vi "PPS_TRAJECTORY_EXECUTE_REL.vi"(8 "Init":bool, 10 "End Relative\nOrientation Deg":dbl, 11 "Gyro Heading\nRAD":dbl) -> (0 "AtReference":bool, 3 "Chassis Velocity Target SI":T7 {"vOmega" format="%10.3f"; "vY" format="%10.3f"; "vX" format="%10.3f"})   [LabVIEW 2019]
uses:
  <vilib>/Rock Robotics/WPI/ThirdParty/JAS_Junk/TrajLib/Trajectory_Library.lvlib
  PPR_TRAJECTORY_GLOBALS.vi
  <vilib>/Rock Robotics/WPI/ThirdParty/MJansen/PathPlanner/PathPlanner24.lvlib
  <vilib>/Rock Robotics/WPI/ThirdParty/JAS_Junk/TrajLib/TypeDef/CHASSIS_SPEEDS.ctl
  <vilib>/Rock Robotics/WPI/ThirdParty/JAS_Junk/TrajLib/TypeDef/TRANSLATION2D.ctl
  <vilib>/Rock Robotics/WPI/ThirdParty/JAS_Junk/TrajLib/TypeDef/ROTATION2D.ctl
  <vilib>/Rock Robotics/WPI/ThirdParty/MJansen/PathPlanner/TypeDef/PathPlannerTrajectory.ctl
  <vilib>/Rock Robotics/WPI/ThirdParty/MJansen/PathPlanner/TypeDef/PathPlannerTrajectoryState.ctl
  <vilib>/Rock Robotics/WPI/ThirdParty/MJansen/PathPlanner/TypeDef/PathPlannerPathConstraints.ctl
panel:
  out "PathPlannerTrajectory":T1 {"States"."TargetHolonomicRotation"."SIN" format="%13.4f"; "States"."TargetHolonomicRotation"."COS" format="%13.4f"; "States"."TargetHolonomicRotation"."VALUE" format="%13.4f"; "States"."Heading"."SIN" format="%13.4f"; "States"."Heading"."COS" format="%13.4f"; "States"."Heading"."VALUE" format="%13.4f"; "States"."PositionMeters"."Y" format="%14.3f"; "States"."PositionMeters"."X" format="%14.3f"}
  in  "Robot Params":T6={"Max Module Speed M/S"=3.2, "Drive Base Radius M"=0.6}
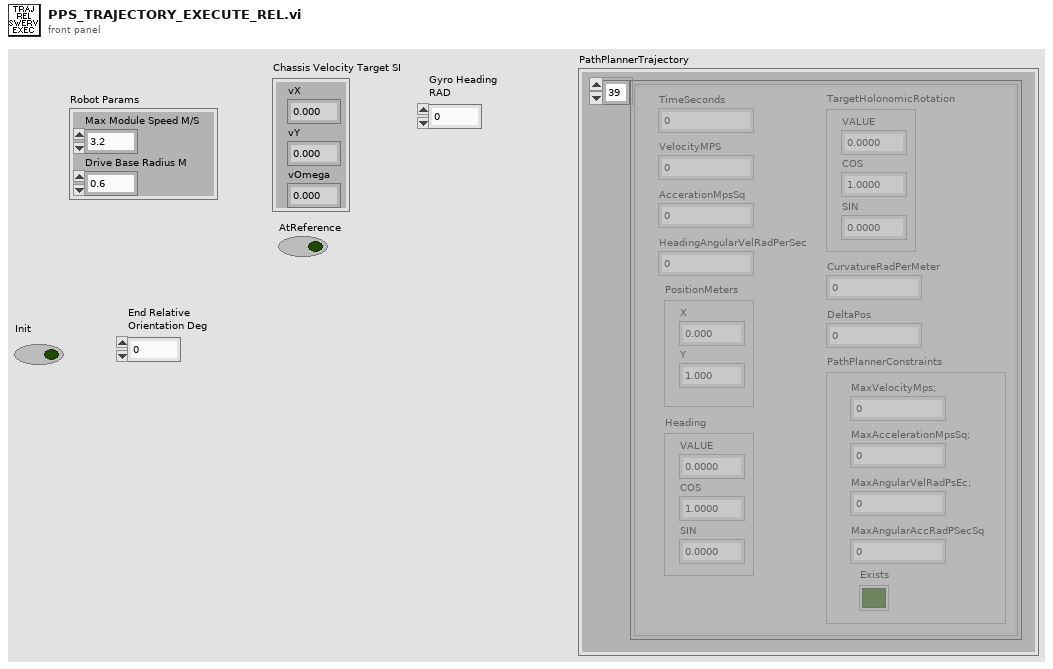
[diagram p1: front panel]
types:
  T1 = typedef "PathPlanner24.lvlib/PathPlannerTrajectory.ctl" = cluster{"States":T2[]}
  T2 = typedef "PathPlanner24.lvlib/PathPlannerTrajectoryState.ctl" = cluster{"TimeSeconds":dbl, "VelocityMPS":dbl, "AccerationMpsSq":dbl, "HeadingAngularVelRadPerSec":dbl, "PositionMeters":T3, "Heading":T4, "TargetHolonomicRotation":T4, "CurvatureRadPerMeter":dbl, "PathPlannerConstraints":T5, "DeltaPos":dbl}
  T3 = typedef "Trajectory_Library.lvlib/TRANSLATION2D.ctl" = cluster{"X":dbl, "Y":dbl}
  T4 = typedef "Trajectory_Library.lvlib/ROTATION2D.ctl" = cluster{"VALUE":dbl, "COS":dbl, "SIN":dbl}
  T5 = typedef "PathPlanner24.lvlib/PathPlannerPathConstraints.ctl" = cluster{"MaxVelocityMps;":dbl, "MaxAccelerationMpsSq;":dbl, "MaxAngularVelRadPsEc;":dbl, "MaxAngularAccRadPSecSq":dbl, "Exists":bool}
  T6 = cluster{"Max Module Speed M/S":dbl, "Drive Base Radius M":dbl}
  T7 = typedef "Trajectory_Library.lvlib/CHASSIS_SPEEDS.ctl" = cluster{"vX":dbl, "vY":dbl, "vOmega":dbl}
  T8 = typedef "Trajectory_Library.lvlib/DIFF_DRIVE_KINEMATICS.ctl" = cluster{"TrackWidth_Meters":dbl}
  T9 = typedef "Trajectory_Library.lvlib/POSE2D.ctl" = cluster{"TRANSLATION":T3, "ROTATION":T4}
  T10 = typedef "Trajectory_Library.lvlib/PID_TUNING.ctl" = cluster{"Kp":dbl, "Ki":dbl, "Kd":dbl, "MaximumIntegral":dbl, "MinimumIntegral":dbl}
  T11 = typedef "Trajectory_Library.lvlib/PROFILED_PID_CONTROLLER.ctl" = cluster{"Controller":T12, "Goal":T13, "Setpoint":T13, "Constraint":T14}
  T12 = typedef "Trajectory_Library.lvlib/PID_CONTROLLER.ctl" = cluster{"Kp":dbl, "Ki":dbl, "Kd":dbl, "Period":dbl, "Max_Integral":dbl, "Min_Integral":dbl, "Max_Input":dbl, "Min_Input":dbl, "Continuous":bool, "PositionError":dbl, "VelocityError":dbl, "PrevError":dbl, "TotalError":dbl, "PositionTolerance":dbl, "VelocityTolerance":dbl, "SetPoint":dbl, "Kf":dbl, "Prev_Deriv":dbl, "Prev_Deriv 2":dbl, "DerivativeFilter":bool, "Min_Output":dbl, "Max_Output":dbl, "Prev_F_P":dbl, "Prev_F_P_2":dbl, "AntiWindupActive":bool, "Measurement":dbl}
  T13 = typedef "Trajectory_Library.lvlib/TRAPEZOID_PROFILE_STATE.ctl" = cluster{"Position":dbl, "Velocity":dbl}
  T14 = typedef "Trajectory_Library.lvlib/TRAPEZOID_PROFILE_CONSTRAINT.ctl" = cluster{"MaxVelocity":dbl, "MaxAcceleration":dbl}
  T15 = typedef "Trajectory_Library.lvlib/HOLONOMIC_PACK_TUNING.ctl" = cluster{"X PID Tuning":T10, "Y PID Tuning":T10, "thetaProfiledPID_CTRL":T11}
  T16 = typedef "Trajectory_Library.lvlib/HOLONOMIC_DRV_CTRL.ctl" = cluster{"poseTolerance":T9, "poseError":T9, "Enabled":bool, "PID_xCtrl":T12, "PID_yCtrl":T12, "PROF_PID_thetaCtrl":T11, "RotationError":T4, "FirstRun":bool}
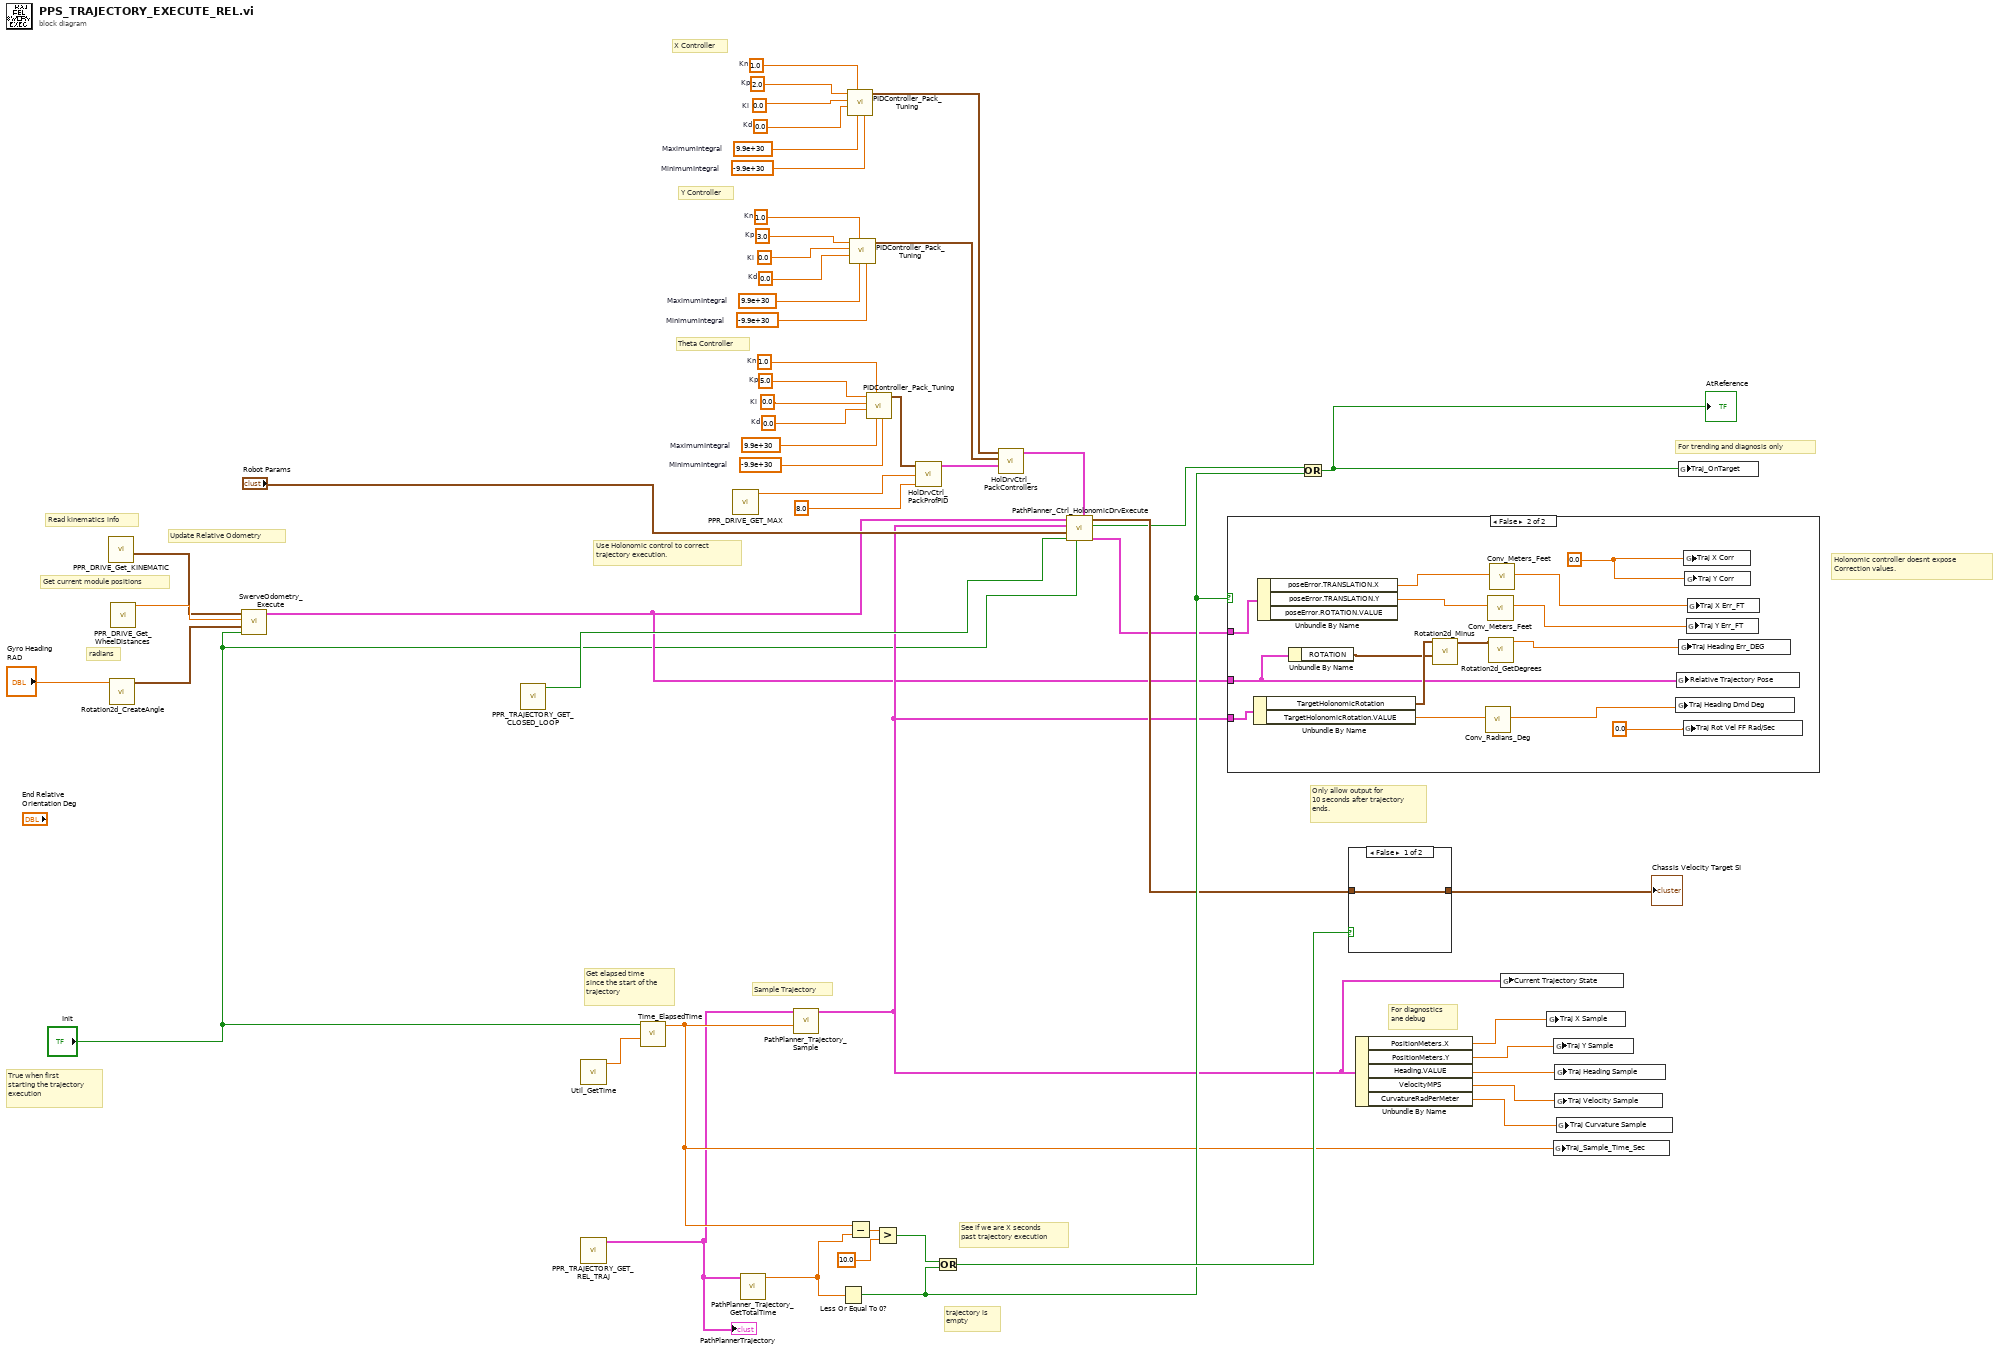
[diagram p0: block diagram]
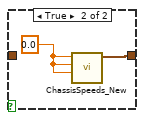
[diagram p3: hidden frame]
diagram:
  w26 = 1.0  # Kn
  w29 = 5.0  # Kp
  w38 = 0.0  # Ki
  w39 = 0.0  # Kd
  w40 = 9.9e+30  # MaximumIntegral
  w41 = -9.9e+30  # MinimumIntegral
  w24 = 1.0  # Kn
  w27 = 2.0  # Kp
  w30 = 0.0  # Ki
  w31 = 0.0  # Kd
  w32 = 9.9e+30  # MaximumIntegral
  w33 = -9.9e+30  # MinimumIntegral
  w25 = 1.0  # Kn
  w28 = 3.0  # Kp
  w34 = 0.0  # Ki
  w35 = 0.0  # Kd
  w36 = 9.9e+30  # MaximumIntegral
  w37 = -9.9e+30  # MinimumIntegral
  # "Get current module positions"
  # "Update Relative Odometry"
  # "Read kinematics info"
  # "radians"
  # "trajectory is \nempty"
  # "Theta Controller"
  # "Y Controller"
  # "X Controller"
  # "True when first\nstarting the trajectory\nexecution"
  # "Get elapsed time\nsince the start of the\ntrajectory"
  # "Holonomic controller doesnt expose\nCorrection values."
  # "Use Holonomic control to correct\ntrajectory execution."
  # "For trending and diagnosis only"
  # "For diagnostics\nane debug"
  # "Sample Trajectory"
  # "See if we are X seconds \npast trajectory execution"
  # "Only allow output for\n10 seconds after trajectory\nends."
  n1 = call "PPR_DRIVE_Get_KINEMATIC.vi"() -> ("out DIFF_DRIVE_KINEMATICS"=w4:T8)  [unwired: 11 in]
  n2 = call <vilib>:"Rotation2d_CreateAngle.vi"("Angle"="Gyro Heading\nRAD") -> ("ROTATION"=w6:T4)  [unwired: 10 in]
  n3 = call "PPR_DRIVE_Get_WheelDistances.vi"() -> ("Left Wheel Dist M"=w5:dbl)  [unwired: 10 in, 1 out]
  n4 = call <vilib>:"SwerveOdometry_Execute.vi"("Init"="Init", "Rotation"=w6, "Swerve Module Positions"=w5, "SWERVE_DRIVE_KINEMATICS"=w4) -> ("Current Pose"=w3:T9)  [unwired: 5 in, 2 out]
  n5 = call "PPR_TRAJECTORY_GET_CLOSED_LOOP.vi"() -> ("AUTO_CLOSED_LOOP"=w15:bool)  [unwired: 11 in]
  n6 = call <vilib>:"Util_GetTime.vi"() -> ("FPGA_Time_Seconds"=w50:dbl)  [unwired: 9 in, 2 out]
  n7 = call "PPR_TRAJECTORY_GET_REL_TRAJ.vi"() -> ("Relative_Trajectory"=w7:T1)  [unwired: 11 in]
  "PathPlannerTrajectory" <- w7
  n8 = call <vilib>:"Time_ElapsedTime.vi"("PassthroughTime_SEC"=w50, "Reset"="Init") -> ("Elapsed Time Sec"=w17:dbl)  [unwired: 9 in]
  n9 = call "PPR_DRIVE_GET_MAX.vi"() -> ("Max Wheel Vel (Meter/Sec)"=w8:dbl)  [unwired: 10 in, 1 out]
  n10 = call <vilib>:"PathPlanner_Trajectory_GetTotalTime.vi"("PathPlannerTrajectory"=w7) -> ("TotalTimeSeconds"=w12:dbl)  [unwired: 10 in]
  n11 = call <vilib>:"PathPlanner_Trajectory_Sample.vi"("Time"=w17, "PathPlannerTrajectory"=w7) -> ("PathPlannerState"=w9:T2)  [unwired: 9 in]
  n12 = Less Or Equal To 0?(x=w12) -> (x <= 0?=w18:bool)
  n13 = call <vilib>:"PIDController_Pack_Tuning.vi"("MinimumIntegral"=w33, "MaximumIntegral"=w32, "Kn"=w24, "Kd"=w31, "Ki"=w30, "Kp"=w27) -> ("PID Tuning"=w42:T10)  [unwired: 5 in]
  n14 = Subtract(x=w17, y=w12) -> (x-y=w53:dbl)
  n15 = call <vilib>:"PIDController_Pack_Tuning.vi"("MinimumIntegral"=w37, "MaximumIntegral"=w36, "Kn"=w25, "Kd"=w35, "Ki"=w34, "Kp"=w28) -> ("PID Tuning"=w43:T10)  [unwired: 5 in]
  n16 = call <vilib>:"PIDController_Pack_Tuning.vi"("MinimumIntegral"=w41, "MaximumIntegral"=w40, "Kn"=w26, "Kd"=w39, "Ki"=w38, "Kp"=w29) -> ("PID Tuning"=w23:T10)  [unwired: 5 in]
  n17 = Greater?(x=w53, y=10.0) -> (0:w21:bool)
  n18 = call <vilib>:"HolDrvCtrl_PackProfPID.vi"("Max Accel"=8.0, "Max Speed"=w8, "Theta PID Tuning"=w23) -> ("Theta PID CONTROLLER"=w44:T11)  [unwired: 8 in]
  n19 = Or(x=w21, y=w18) -> (x .or. y?=w20:bool)
  n20 = call <vilib>:"HolDrvCtrl_PackControllers.vi"("thetaProfiledPID_CTRL"=w44, "Y PID Tuning"=w43, "X PID Tuning"=w42) -> ("HOLONOMIC_CTRL_PACK_TUNING"=w16:T15)  [unwired: 8 in]
  n21 = call <vilib>:"PathPlanner_Ctrl_HolonomicDrvExecute.vi"("HOLONOMIC_CTRL_PACK_TUNING"=w16, "Reset"="Init", "Enabled"=w15, "Robot Parameters"="Robot Params", "PathPlannerState"=w9, "Current Pose SI"=w3) -> ("outHOLONOMIC_DRV_CTRL"=w10:T16, "At Reference"=w13:bool, "calcChassisSpeed"=w14:T7)  [unwired: 2 in, 1 out]
  n22 = case shown="False" w18 {
    tunnel: w3 -> [_ w57]
    tunnel: w10 -> [_ w64]
    tunnel: w9 -> [_ w61]
    frame True {
    }
    frame False {
      w68 = 0.0 ("Y Corr")
      n23 = Unbundle By Name(w61) -> ("TargetHolonomicRotation"=w58:T4, "TargetHolonomicRotation.VALUE"=w60:dbl)
      n24 = Unbundle By Name(w64) -> ("poseError.TRANSLATION.X"=w63:dbl, "poseError.TRANSLATION.Y"=w62:dbl)  [unwired: 1 out]
      n25 = Unbundle By Name(w57) -> ("ROTATION"=w56:T4)
      n26 = call <vilib>:"Rotation2d_Minus.vi"("other ROTATION"=w56, "in ROTATION"=w58) -> ("out ROTATION"=w55:T4)  [unwired: 9 in]
      n27 = call <vilib>:"Conv_Radians_Deg.vi"("Radians"=w60) -> ("Degrees"=w59:dbl)  [unwired: 10 in]
      n28 = call <vilib>:"Conv_Meters_Feet.vi"("Meters"=w62) -> ("Feet"=w67:dbl)  [unwired: 10 in]
      n29 = call <vilib>:"Rotation2d_GetDegrees.vi"("in ROTATION"=w55) -> ("AngleDegrees"=w54:dbl)  [unwired: 10 in]
      n30 = call <vilib>:"Conv_Meters_Feet.vi"("Meters"=w63) -> ("Feet"=w66:dbl)  [unwired: 10 in]
      n31 = global write "PPR_TRAJECTORY_GLOBALS.vi" "Traj Heading Dmd Deg"(w59) -> ()
      n32 = global write "PPR_TRAJECTORY_GLOBALS.vi" "Relative Trajectory Pose"(w57) -> ()
      n33 = global write "PPR_TRAJECTORY_GLOBALS.vi" "Traj Heading Err_DEG"(w54) -> ()
      n34 = global write "PPR_TRAJECTORY_GLOBALS.vi" "Traj Rot Vel FF Rad/Sec"(0.0 ("Traj Heading Dmd Deg")) -> ()
      n35 = global write "PPR_TRAJECTORY_GLOBALS.vi" "Traj X Corr"(w68) -> ()
      n36 = global write "PPR_TRAJECTORY_GLOBALS.vi" "Traj Y Corr"(w68) -> ()
      n37 = global write "PPR_TRAJECTORY_GLOBALS.vi" "Traj Y Err_FT"(w67) -> ()
      n38 = global write "PPR_TRAJECTORY_GLOBALS.vi" "Traj X Err_FT"(w66) -> ()
    }
  }
  n39 = Or(x=w13, y=w18) -> (x .or. y?=w19:bool)
  "AtReference" <- w19
  n40 = case shown="False" w20 {
    tunnel: w14 -> [w69 _]
    tunnel: [w69 w70] -> w51
    frame False {
    }
    frame True {
      w71 = 0.0 ("vX")
      n41 = call <vilib>:"ChassisSpeeds_New.vi"("vAngular"=w71, "vY"=w71, "vX"=w71) -> ("CHASSIS"=w70:T7)  [unwired: 8 in]
    }
  }
  "Chassis Velocity Target SI" <- w51
  n42 = Unbundle By Name(w9) -> ("PositionMeters.X"=w49:dbl, "PositionMeters.Y"=w48:dbl, "Heading.VALUE"=w47:dbl, "VelocityMPS"=w46:dbl, "CurvatureRadPerMeter"=w45:dbl)
  n43 = global write "PPR_TRAJECTORY_GLOBALS.vi" "Current Trajectory State"(w9) -> ()
  n44 = global write "PPR_TRAJECTORY_GLOBALS.vi" "Traj X Sample"(w49) -> ()
  n45 = global write "PPR_TRAJECTORY_GLOBALS.vi" "Traj_Sample_Time_Sec"(w17) -> ()
  n46 = global write "PPR_TRAJECTORY_GLOBALS.vi" "Traj Y Sample"(w48) -> ()
  n47 = global write "PPR_TRAJECTORY_GLOBALS.vi" "Traj Heading Sample"(w47) -> ()
  n48 = global write "PPR_TRAJECTORY_GLOBALS.vi" "Traj Velocity Sample"(w46) -> ()
  n49 = global write "PPR_TRAJECTORY_GLOBALS.vi" "Traj Curvature Sample"(w45) -> ()
  n50 = global write "PPR_TRAJECTORY_GLOBALS.vi" "Traj_OnTarget"(w19) -> ()
